vi "get pythonw pid.vi"(3 "error in (no error)":errorcluster) -> (0 "error out":errorcluster, 1 "PIDs":i32[](array[numeric]))   [LabVIEW 2018]
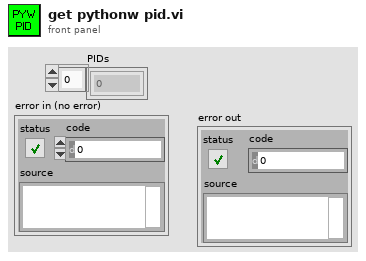
[diagram p1: front panel]
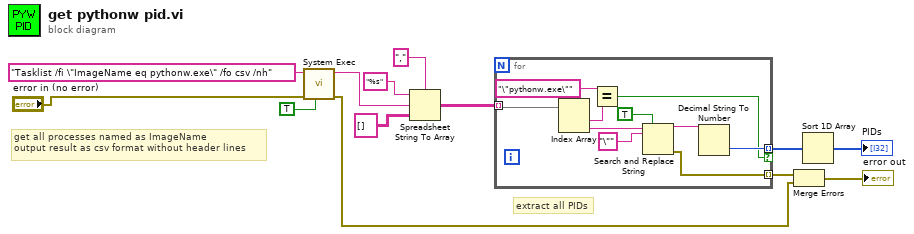
[diagram p0: block diagram]
diagram:
  # "extract all PIDs"
  # "get all processes named as ImageName\noutput result as csv format without header lines"
  n1 = call <vilib>:"System Exec.vi"("run minimized? (F)"=TRUE, "error in (no error)"="error in (no error)", "command line"="Tasklist /fi \"ImageName eq pythonw.exe\" /fo csv /nh") -> ("error out"=w4:errorcluster, "standard output"=w9:string)  [unwired: 5 in, 2 out]
  n2 = Spreadsheet String To Array(delimiter (Tab)=",", format string="%s", spreadsheet string=w9, array type (2D Dbl)=string[][] []) -> (array=w12:string[][])
  n3 = for {
    tunnel: w12 -> [w23] mode=indexing
    tunnel: [w18] -> w2 mode=indexing if=w15
    tunnel: [w14] -> w5 mode=indexing
    n4 = Index Array(array=w23) -> (element #1=w17:string, element #2=w22:string)  [unwired: 2 in]
    n5 = Equal?(x="\"pythonw.exe\"", y=w17) -> (x = y?=w15:bool)
    n6 = Search and Replace String(replace all?=TRUE ("replace all? (F)"), input string=w22, search string="\"") -> (result string=w19:string, error out=w14:errorcluster)  [unwired: 5 in, 2 out]
    n7 = Decimal String To Number(string=w19) -> (number=w18:i32)  [unwired: 2 in, 1 out]
  }
  n8 = Merge Errors(w5, w4) -> (→"error out":errorcluster)
  n9 = Sort 1D Array(array=w2) -> (sorted array=→"PIDs":i32[])
